vi "Enqueue Message (Single).vi"(6 "Priority Message? (F)":bool, 8 "error in (no error)":errorcluster, 9 "Message Data":variant, 10 "test sequence":T1 caption="Enum", 11 "Message Queue":refnum<queue>) -> (0 "error out":errorcluster, 3 "dup Message Queue":refnum<queue>)   [LabVIEW 2021, in "RMU Message Queue.lvlib"]
doc: "For a regular message, enqueue the message. For a priority message, enqueue it at the front of the queue."
uses:
  RMU Message Queue.lvlib
  Message Cluster.ctl
  controls/developer_test sequence.ctl
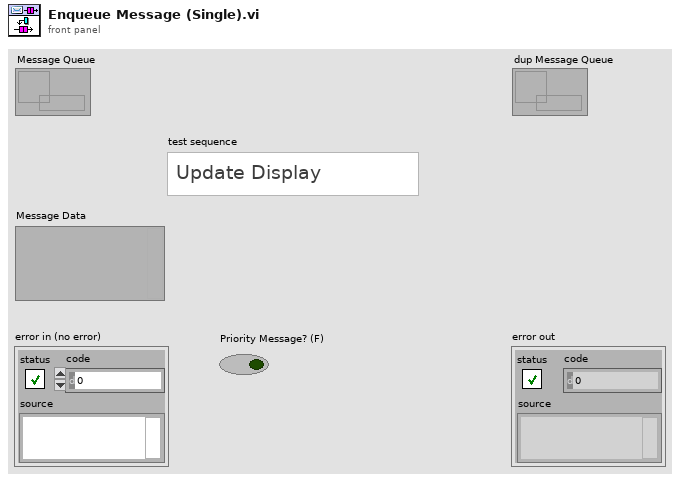
[diagram p1: front panel]
types:
  T1 = typedef "developer_test sequence.ctl" = enum16{"Update Display", "User Login", "Admin", "Initialise", "Init Devices", "Idle State", "test steup", "Abort", "Start Display Board Auto Testing", "Scan Barcode", "Checking TEMP at Thermistor 1", "Checking TEMP at Thermistor 2", "Checking TEMP at Thermistor 3", "Checking TEMP at Thermistor 4 (Ambient)", "Voltage Health Check", "INSULATION Resistance test (Baseplate to Negative)", "INSULATION Resistance test (Baseplate to Positive)", "WELD Resistance Test", "Stop Display Board Auto Testing", "All Pass", "Fail", "Report", "Error", "Confirm Quit", "Exit"}
  T2 = typedef "RMU Message Queue.lvlib/Message Cluster.ctl" = cluster{"test sequence":T1, "Message Data":variant}
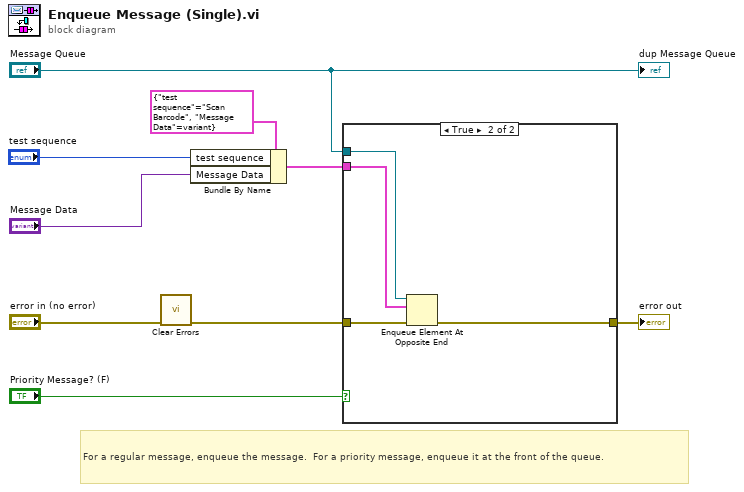
[diagram p0: block diagram]
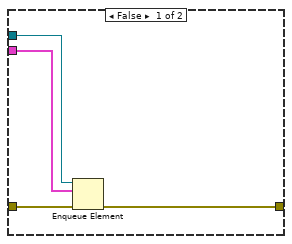
[diagram p2: hidden frame]
diagram:
  # "For a regular message, enqueue the message.  For a priority message, enqueue it at the front of the queue."
  n1 = call <vilib>:"Clear Errors.vi"("error in (no error)"="error in (no error)") -> ("error out"=w1:errorcluster)  [unwired: 5 in, 1 out]
  n2 = Bundle By Name(cluster=T2 {"test sequence"=enum."Scan Barcode", "Message Data"=variant} ("Message Cluster"), "test sequence"="test sequence", "Message Data"="Message Data") -> (w4:T2)
  n3 = case shown="True" "Priority Message? (F)" {
    tunnel: w1 -> [w13 w17]
    tunnel: [w12 w16] -> w6
    tunnel: "Message Queue" -> [w11 w15]
    tunnel: w4 -> [w10 w14]
    frame False {
      n4 = Enqueue Element(queue=w11, element=w10, error in (no error)=w13) -> (error out=w12:errorcluster)  [unwired: 1 in, 2 out]
    }
    frame True {
      n5 = Enqueue Element At Opposite End(queue=w15, element=w14, error in (no error)=w17) -> (error out=w16:errorcluster)  [unwired: 1 in, 2 out]
    }
  }
  "error out" <- w6
  "dup Message Queue" <- "Message Queue"
